vi "PCmain.vi"() -> ()   [LabVIEW 2019]
uses:
  <vilib>/OSIsoft/Academic Hub Toolkit/support/ACS_Asset.ctl
  <vilib>/OSIsoft/Academic Hub Toolkit/support/ACS_Types.ctl
  <vilib>/OSIsoft/Academic Hub Toolkit/support/AssetProperties.ctl
  <vilib>/OSIsoft/Academic Hub Toolkit/support/DataTypes.ctl
  <vilib>/Platform/TimedLoop/XDataNode/timing_clust.ctl
  <vilib>/Platform/TimedLoop/XDataNode/nitl_modes.ctl
  <vilib>/Platform/TimedLoop/XDataNode/wakeup.ctl
  <vilib>/Platform/TimedLoop/XDataNode/XDataNode.xnode
  <vilib>/Platform/TimedLoop/XDataNode/XDNodeRunTimeDep.lvlib
  <vilib>/OSIsoft/Academic Hub Toolkit/support/ACS_Support.lvlib
panel:
  out "OMFListener status":string
  out "error out":errorcluster
  in  "ACS Info":T1={"OMFListener URL"="http://localhost:6008/ingress/messages", "Configuration\n  Init | Run"=TRUE, "Configuration filename"="Sample_array_data.ini", "Type"=FALSE, "Container"=FALSE, "Data"=FALSE, "ACS Asset"={"Asset Properties"=[], "Asset Attributes"=[], "Asset Name"="", "Template Name"=""}, "Asset_ID"=0, "Offline"=FALSE, "Error"=FALSE}
  in  "RECORD \nto Cloud":bool
  out "ON BOTTOM":bool
  in  "Zero \nWOB":bool
  out "DiffP":dbl(knob) scale=0.0..3000.0
  out "WOB":dbl(knob) scale=0.0..10000.0
  out "Blk Pos":dbl format="%.3f"
  out "ROP":dbl
  out "Block Position":cluster{dbl, dbl, dbl[]}(graph)
  out "Pin":dbl format="%.1f"
  out "Pout":dbl format="%#.1f"
  out "DeltaP":dbl format="%.1f"
  out "Differential Pressure":cluster{dbl, dbl, dbl[]}(graph)
  out "rpm":dbl
  out "RPM":dbl(knob) scale=0.0..2000.0
  out "Rotational Speed":cluster{dbl, dbl, dbl[]}(graph)
  out "Load 2":dbl format="%.1f"
  out "Load 1":dbl format="%.1f"
  out "WOB":dbl format="%.1f"
  out "Time":timestamp
  out "Recording":bool
  out "Torque":dbl
  in  "RECORD":bool
  out "Weight-on-Bit":cluster{dbl, dbl, dbl[][]}(graph)
  # "ft/hr"
  # "ft"
  # "ft/lbf"
  # "OMF:"
  # "Hub Status:"
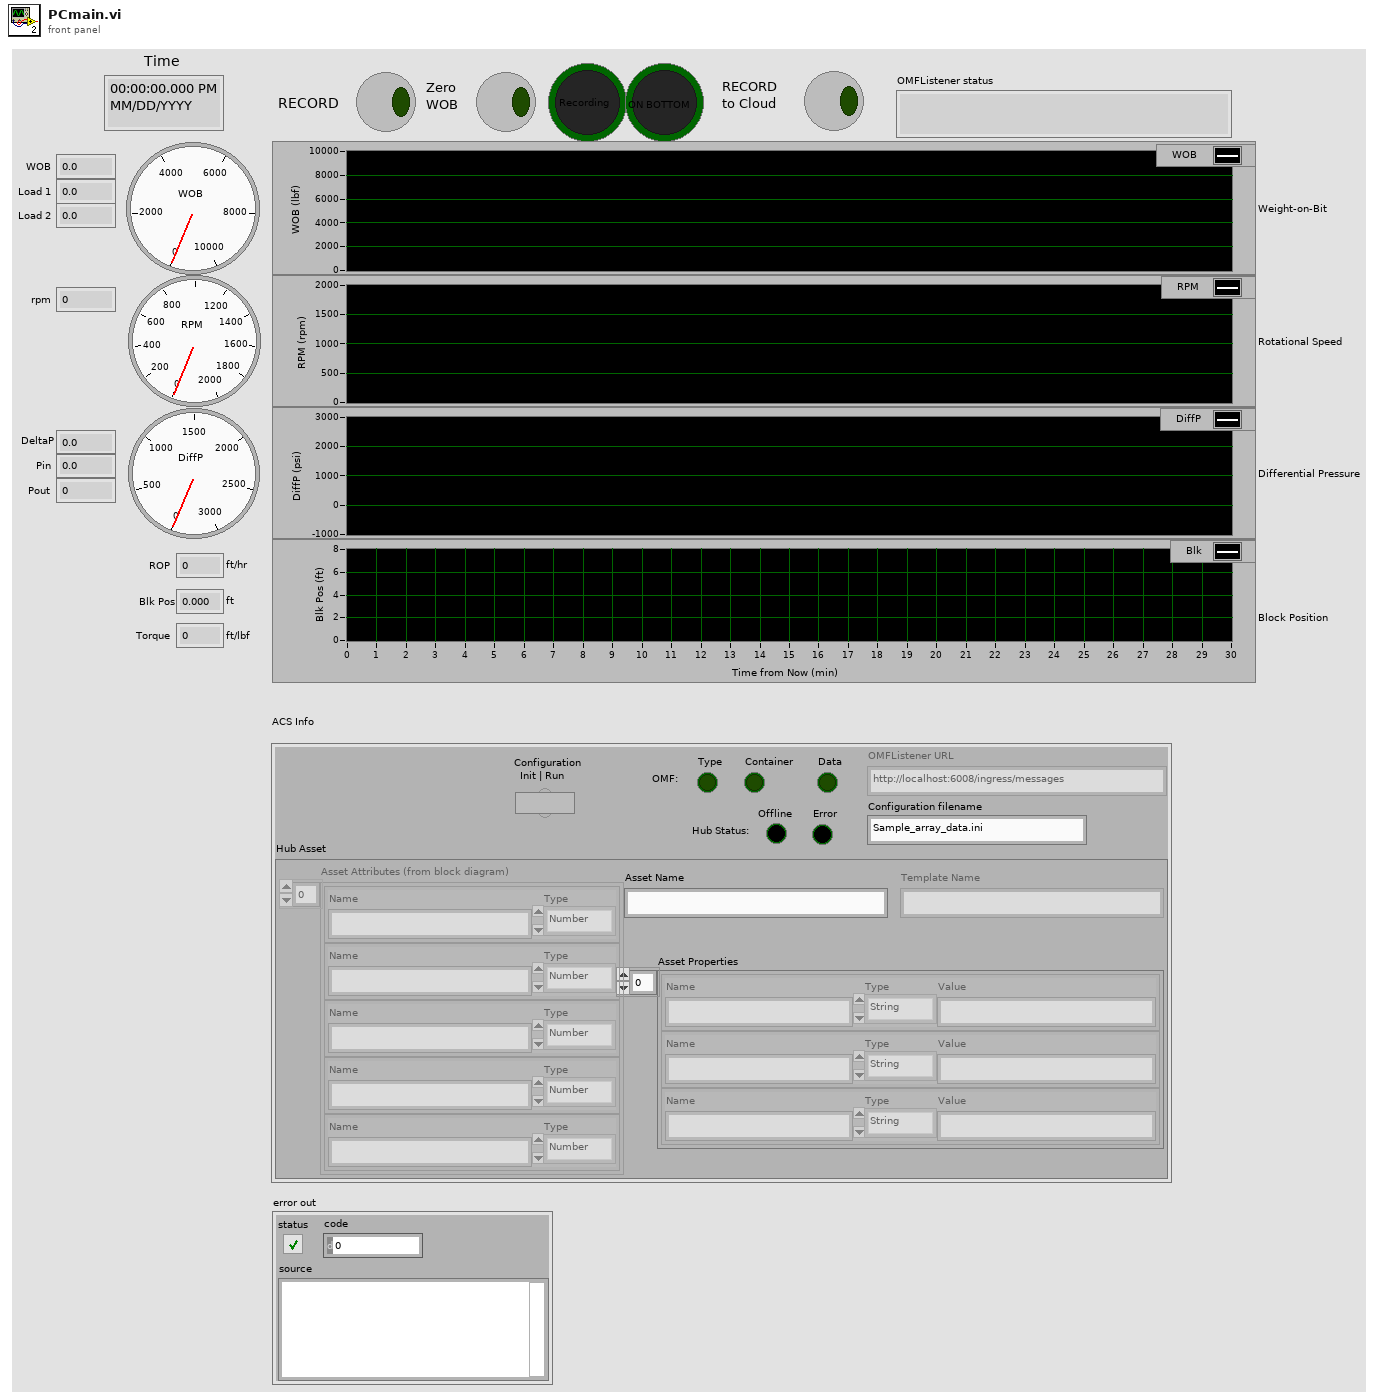
[diagram p1: front panel]
types:
  T1 = typedef "ACS_Support.lvlib/ACS_Asset.ctl" = cluster{"OMFListener URL":string, "Configuration\n  Init | Run":bool, "Configuration filename":string, "Type":bool, "Container":bool, "Data":bool, "ACS Asset":T2, "Asset_ID":u8, "Offline":bool, "Error":bool}
  T2 = typedef "ACS_Support.lvlib/ACS_Types.ctl" = cluster{"Asset Properties":T3, "Asset Attributes":T4, "Asset Name":string, "Template Name":string}
  T3 = typedef "ACS_Support.lvlib/AssetProperties.ctl" = cluster{"Name":string, "Type":enum16{"String", "Number"}, "Value":string}[]
  T4 = typedef "ACS_Support.lvlib/DataTypes.ctl" = cluster{"Name":string, "Type":enum16{"Number", "String"}}[]
  T5 = typedef "ACS_Support.lvlib/ACPI_Session.ctl" = cluster{"client handle out":T6, "stream_id_for_sending_values":string, "ACS Info":T1, "PI-Data":T7, "ACS Asset ref":refnum<vi>, "Main VI ref":refnum<vi>, "Message Queue":refnum<queue>, "Timestamp":timestamp}
  T6 = typedef "LabVIEWHTTPClient.lvlib/ClientHandle.ctl" = refnum<k1>
  T7 = typedef "ACS_Support.lvlib/PI-Data.ctl" = cluster{"PI-DVNT":variant, "PI-Values":variant, "PI-error":bool}
  T8 = typedef "XDNodeRunTimeDep.lvlib/timing_clust.ctl" = cluster{"Expected End [f-1]":u64, "Actual End [f-1]":u64, "Finished Late? [f-1]":bool, "Expected End [i-1]":u64, "Actual End [i-1]":u64, "Finished Late? [i-1]":bool, "Expected Start [i]":u64, "Actual Start [i]":u64, "Expected Start [f]":u64, "Actual Start [f]":u64, "Source Name":string, "Structure Name":string, "Period":i64, "Deadline":i64, "Offset":i64, "Start":i64, "Priority":i32, "Timeout":i32, "Mode":T9, "Wakeup Reason":T10, "Error":errorcluster, "Source Type":string, "Secondary Source Type":string, "Global End Time":u64, "Global Start Time":u64, "Frame Duration":u64, "Iteration Duration":u64, "Assigned CPU":i32, "I/O Scan Engine Mode":u32}
  T9 = typedef "XDNodeRunTimeDep.lvlib/nitl_modes.ctl" = enum32{"No Change", "Process missed periods, maintain original phase", "Discard missed periods, maintain original phase", "Process missed periods, ignore original phase", "Discard missed periods, ignore original phase"}
  T10 = typedef "XDNodeRunTimeDep.lvlib/wakeup.ctl" = enum32{"Normal", "Aborted", "Asynchronous wakeup", "Timing source error", "Timed loop error", "Timeout"}
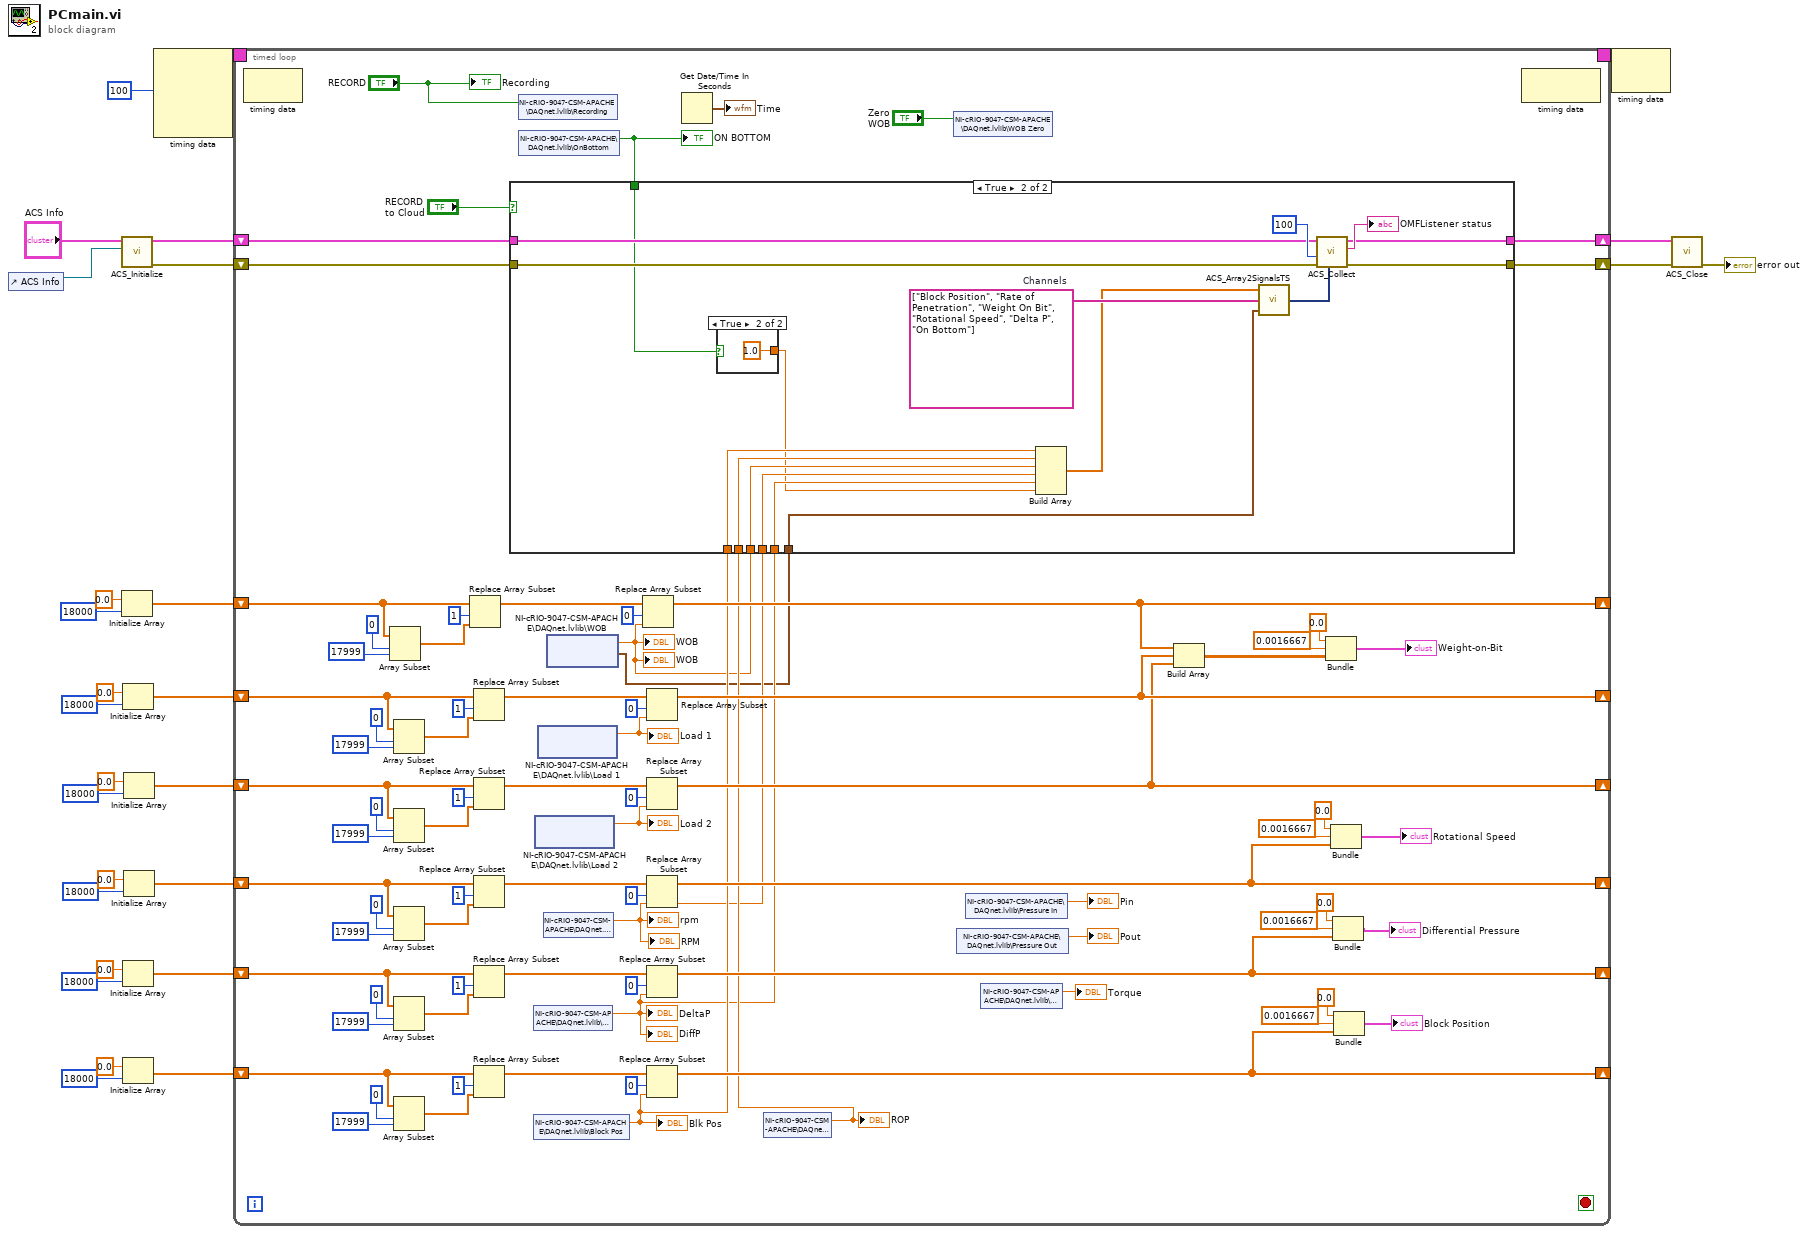
[diagram p0: block diagram]
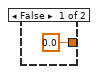
[diagram p3: hidden frame]
diagram:
  n1 = control-ref of="ACS Info"() -> (w6:refnum<vi>)
  n2 = call <vilib>:"ACS_Initialize.vi"("ACS Asset ref"=w6, "ACS Asset"="ACS Info") -> ("error out"=w5:errorcluster, "ACPI Session out"=w4:T5)  [unwired: 4 in, 1 out]
  n3 = Initialize Array(0.0 ("element"), 18000 ("dimension size")) -> (w23:dbl[])
  n4 = Initialize Array(0.0 ("element"), 18000 ("dimension size")) -> (w20:dbl[])
  n5 = Initialize Array(0.0 ("element"), 18000 ("dimension size")) -> (w8:dbl[])
  n6 = Initialize Array(0.0 ("element"), 18000 ("dimension size")) -> (w9:dbl[])
  n7 = Initialize Array(0.0 ("element"), 18000 ("dimension size")) -> (w17:dbl[])
  n8 = Initialize Array(0.0 ("element"), 18000 ("dimension size")) -> (w14:dbl[])
  n9 = node-c288(i64 100 ("Period")) -> (w28:T8)  [unwired: 3 in]
  n10 = timed-loop {
    timing: w28 -> [_]
    timing-out: [_] -> w27
    shift-right: [w87] -> _
    shift-left: w23 -> [w98]
    shift-right: [w86] -> _
    shift-left: w20 -> [w88]
    shift-right: [w75] -> _
    shift-left: w17 -> [w76]
    shift-right: [w65] -> _
    shift-left: w14 -> [w68]
    shift-right: [w42] -> _
    shift-left: w8 -> [w50]
    shift-right: [w43] -> _
    shift-left: w9 -> [w51]
    shift-right: [w37] -> w3
    shift-left: w5 -> [w36]
    shift-right: [w38] -> w2
    shift-left: w4 -> [w39]
    stop <- _ stop-if-true
    n11 = node-c288() -> ()  [unwired: 1 in, 1 out]
    n12 = Array Subset(array=w98, index=0, length=17999) -> (w102:dbl[])
    n13 = Array Subset(array=w88, index=0, length=17999) -> (w92:dbl[])
    n14 = Array Subset(array=w76, index=0, length=17999) -> (w81:dbl[])
    n15 = Array Subset(array=w68, index=0, length=17999) -> (w72:dbl[])
    n16 = Array Subset(array=w50, index=0, length=17999) -> (w54:dbl[])
    n17 = Array Subset(array=w51, index=0, length=17999) -> (w61:dbl[])
    n18 = Replace Array Subset(array=w98, new element=w102, index=1) -> (w103:dbl[])
    n19 = Replace Array Subset(array=w88, new element=w92, index=1) -> (w93:dbl[])
    n20 = Replace Array Subset(array=w76, new element=w81, index=1) -> (w82:dbl[])
    n21 = Replace Array Subset(array=w68, new element=w72, index=1) -> (w73:dbl[])
    n22 = Replace Array Subset(array=w50, new element=w54, index=1) -> (w53:dbl[])
    n23 = Replace Array Subset(array=w51, new element=w61, index=1) -> (w62:dbl[])
    n24 = shared-variable "NI-cRIO-9047-CSM-APACHE\\DAQnet.lvlib\\Recording"("RECORD") -> ()  [unwired: 1 in, 1 out]
    n25 = shared-variable "NI-cRIO-9047-CSM-APACHE\\DAQnet.lvlib\\OnBottom"() -> (w30:bool)  [unwired: 1 in, 1 out]
    "ON BOTTOM" <- w30
    n26 = shared-variable "NI-cRIO-9047-CSM-APACHE\\DAQnet.lvlib\\DeltaP"() -> (w31:dbl)  [unwired: 1 in, 1 out]
    "DiffP" <- w31
    "DeltaP" <- w31
    n27 = shared-variable "NI-cRIO-9047-CSM-APACHE\\DAQnet.lvlib\\Block Pos"() -> (w35:dbl)  [unwired: 1 in, 1 out]
    "Blk Pos" <- w35
    n28 = shared-variable "NI-cRIO-9047-CSM-APACHE\\DAQnet.lvlib\\Load 2"() -> (w77:dbl)  [unwired: 1 in, 2 out]
    "Load 2" <- w77
    n29 = shared-variable "NI-cRIO-9047-CSM-APACHE\\DAQnet.lvlib\\Load 1"() -> (w84:dbl)  [unwired: 1 in, 2 out]
    "Load 1" <- w84
    n30 = shared-variable "NI-cRIO-9047-CSM-APACHE\\DAQnet.lvlib\\RPM"() -> (w32:dbl)  [unwired: 1 in, 1 out]
    "RPM" <- w32
    "rpm" <- w32
    n31 = shared-variable "NI-cRIO-9047-CSM-APACHE\\DAQnet.lvlib\\WOB"() -> (w33:dbl, w29:timestamp)  [unwired: 1 in, 1 out]
    "WOB" <- w33
    "WOB" <- w33
    n32 = Replace Array Subset(array=w103, new element=w33, index=0) -> (w87:dbl[])
    n33 = Replace Array Subset(array=w93, new element=w84, index=0) -> (w86:dbl[])
    n34 = Replace Array Subset(array=w82, new element=w77, index=0) -> (w75:dbl[])
    n35 = Replace Array Subset(array=w73, new element=w32, index=0) -> (w65:dbl[])
    n36 = Replace Array Subset(array=w53, new element=w31, index=0) -> (w42:dbl[])
    n37 = Replace Array Subset(array=w62, new element=w35, index=0) -> (w43:dbl[])
    n38 = Get Date/Time In Seconds() -> (seconds since 1Jan1904=→"Time":timestamp)
    n39 = shared-variable "NI-cRIO-9047-CSM-APACHE\\DAQnet.lvlib\\ROP"() -> (w34:dbl)  [unwired: 1 in, 1 out]
    "ROP" <- w34
    n40 = case shown="True" "RECORD \nto Cloud" {
      tunnel: w39 -> [w111 w124]
      tunnel: [w111 w123] -> w38
      tunnel: [w110 w122] -> w37
      tunnel: w36 -> [w110 w121]
      tunnel: w35 -> [_ w119]
      tunnel: w34 -> [_ w118]
      tunnel: w33 -> [_ w117]
      tunnel: w32 -> [_ w116]
      tunnel: w31 -> [_ w115]
      tunnel: w30 -> [_ w114]
      tunnel: w29 -> [_ w112]
      frame False {
      }
      frame True {
        w128 = string[] ["Block Position", "Rate of Penetration", "Weight On Bit", "Rotational Speed", "Delta P", "On Bottom"]  # Channels
        n41 = case shown="True" w114 {
          tunnel: [0.0 1.0] -> w113
          frame False {
          }
          frame True {
          }
        }
        n42 = Build Array(w119, w118, w117, w116, w115, w113) -> (w120:dbl[])
        n43 = call <vilib>:"ACS_Array2SignalsTS.vi"("Timestamp"=w112, "signal names"=w128, "array"=w120) -> ("signals out"=w127:dynamicdata)
        n44 = call <vilib>:"ACS_Collect.vi"("Signals In"=w127, "error in"=w121, "OMF batch"=100, "ACPI Session in"=w124) -> ("error out"=w122:errorcluster, "OMFListener status"=→"OMFListener status":string, "ACPI Session out"=w123:T5)  [unwired: 1 in, 1 out]
      }
    }
    n45 = shared-variable "NI-cRIO-9047-CSM-APACHE\\DAQnet.lvlib\\WOB Zero"("Zero \nWOB") -> ()  [unwired: 1 in, 1 out]
    n46 = shared-variable "NI-cRIO-9047-CSM-APACHE\\DAQnet.lvlib\\Pressure Out"() -> (→"Pout":dbl)  [unwired: 1 in, 1 out]
    n47 = shared-variable "NI-cRIO-9047-CSM-APACHE\\DAQnet.lvlib\\Pressure In"() -> (→"Pin":dbl)  [unwired: 1 in, 1 out]
    n48 = shared-variable "NI-cRIO-9047-CSM-APACHE\\DAQnet.lvlib\\Torque"() -> (→"Torque":dbl)  [unwired: 1 in, 1 out]
    n49 = Build Array(w87, w86, w75) -> (w85:dbl[][])
    n50 = Bundle(0.0, 0.0016667, w85) -> (→"Weight-on-Bit":cluster{dbl, dbl, dbl[][]})  [unwired: 1 in]
    n51 = Bundle(0.0, 0.0016667, w65) -> (→"Rotational Speed":cluster{dbl, dbl, dbl[]})  [unwired: 1 in]
    n52 = Bundle(0.0, 0.0016667, w42) -> (→"Differential Pressure":cluster{dbl, dbl, dbl[]})  [unwired: 1 in]
    n53 = Bundle(0.0, 0.0016667, w43) -> (→"Block Position":cluster{dbl, dbl, dbl[]})  [unwired: 1 in]
    n54 = node-c288() -> ()  [unwired: 1 in, 1 out]
    "Recording" <- "RECORD"
  }
  n55 = node-c288(w27) -> ()  [unwired: 1 out]
  n56 = call <vilib>:"ACS_Close.vi"("error in (no error)"=w3, "Ref In"=w2) -> ("error out"=→"error out":errorcluster)  [unwired: 9 in]
